vi "UTF-8 To UTF-16.vi"(8 "error in (no error)":errorcluster, 11 "UTF-8":string) -> (0 "error out":errorcluster, 3 "UTF-16":string)   [LabVIEW 2020, in "G-Audio.lvlib"]
doc: "Converts a UTF-8 encoded string to UTF-16 LE using Windows' MultiByteToWideChar() function.\n\nNote: This function only works on Windows. When called from macOS or Linux, the output string will have the same encoding as the input string, and a warning will appear on the error wire."
uses:
  G-Audio.lvlib
  <vilib>/Utility/error.llb/Error Cluster From Error Code.vi
  lib/g_audio_32.dll
panel:
  # "Force Unicode Text is enabled on this string indicator."
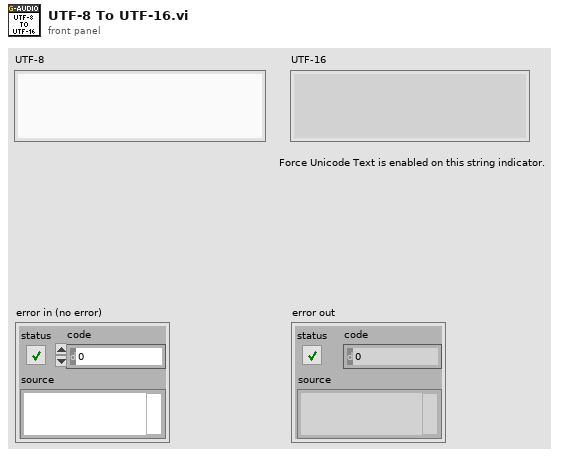
[diagram p1: front panel]
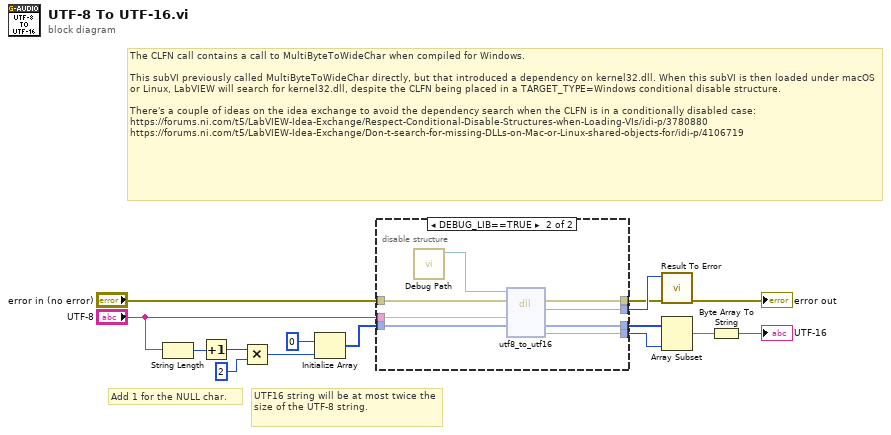
[diagram p0: block diagram]
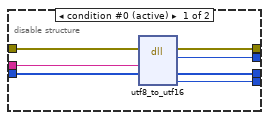
[diagram p2: hidden frame]
diagram:
  # "Add 1 for the NULL char."
  # "The CLFN call contains a call to MultiByteToWideChar when compiled for Windows.\n\nThis subVI previously called MultiByteToWideChar directly, but that introduced a dependency on kernel32.dll. When this subVI is then loaded under macOS or Linux, LabVIEW will search for kernel32.dll, despite the CLFN being placed in a TARGET_TYPE=Windows conditional disable structure.\n\nThere's a couple of ideas on the idea exchange to avoid the dependency search when the CLFN is in a conditionally disabled case:\nhttps://forums.ni.com/t5/LabVIEW-Idea-Exchange/Respect-Conditional-Disable-Structures-when-Loading-VIs/idi-p/3780880\nhttps://forums.ni.com/t5/LabVIEW-Idea-Exchange/Don-t-search-for-missing-DLLs-on-Mac-or-Linux-shared-objects-for/idi-p/4106719"
  # "UTF16 string will be at most twice the size of the UTF-8 string."
  n1 = String Length(string="UTF-8") -> (length=w5:i32)
  n2 = Increment(x=w5) -> (x+1=w4:i32)
  n3 = Multiply(x=w4, y=2) -> (x*y=w3:i32)
  n4 = Initialize Array(u8 0, w3) -> (w9:u8[])
  n5 = disable-structure shown="DEBUG_LIB==TRUE" {
    disable-tunnel: [w22 w30] -> w7
    disable-tunnel: "error in (no error)" -> [w21 w29]
    disable-tunnel: "UTF-8" -> [w17 w25]
    disable-tunnel: [w20 w28] -> w15
    disable-tunnel: w9 -> [w16 w24]
    disable-tunnel: [w19 w27] -> w11
    disable-tunnel: [w18 w26] -> w2
    frame condition #0 (active) {
      n6 = dll-call lib="C:/github/dataflowg/g-audio/src/LabVIEW/G-Audio/lib/g_audio_*.*" fn="utf8_to_utf16"(error in=w21, "utf_string"=w17, "utf16_string"=w16) -> (error out=w22:errorcluster, "result"=w20:i32, "utf16_string"=w19:u8[], "utf16_length"=w18:i32)  [unwired: 4 in, 1 out]
    }
    frame condition #1 {
      n7 = call "Debug Path.vi"() -> ("Debug Path"=w23:path)  [unwired: 11 in]
      n8 = dll-call lib="?" fn="utf8_to_utf16"(path in=w23, error in=w29, "utf_string"=w25, "utf16_string"=w24) -> (error out=w30:errorcluster, "result"=w28:i32, "utf16_string"=w27:u8[], "utf16_length"=w26:i32)  [unwired: 3 in, 1 out]
    }
  }
  n9 = call "Result To Error.vi"("error in (no error)"=w7, "Result Code"=w15) -> ("error out"=→"error out":errorcluster)  [unwired: 9 in]
  n10 = Array Subset(array=w11, length=w2) -> (w10:u8[])  [unwired: 1 in]
  n11 = Byte Array To String(unsigned byte array=w10) -> (string=→"UTF-16":string)
